vi "GetHight.vi"(8 "error in (no error)":errorcluster, 11 "Triangle in":refnum<class "Triangle.lvclass">) -> (0 "error out":errorcluster, 2 "Hight":i16, 3 "Triangle out":refnum<class "Triangle.lvclass">)   [LabVIEW 2021, in "Picture2D.lvlib" / "Triangle.lvclass"]
uses:
  Triangle.lvclass
  Triangle.lvclass/Triangle.ctl
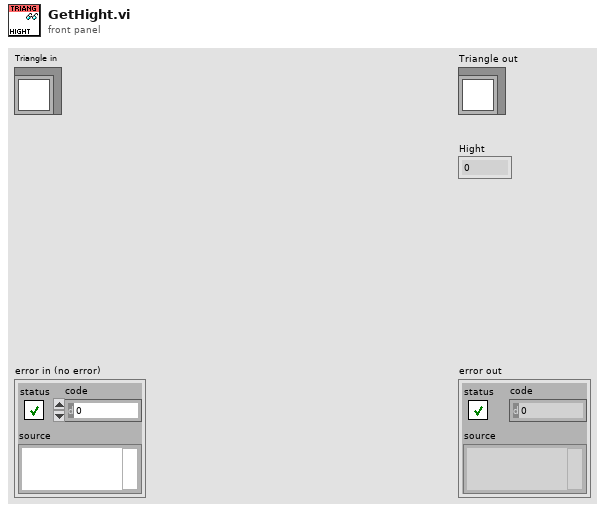
[diagram p1: front panel]
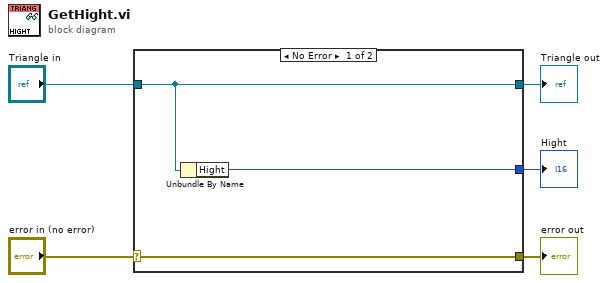
[diagram p0: block diagram]
diagram:
  n1 = case shown="No Error" "error in (no error)" {
    selector: "error in (no error)" -> [w8 w9]
    tunnel: [w8 w9] -> w4
    tunnel: [w7 w10] -> w2
    tunnel: "Triangle in" -> [w7 w10]
    tunnel: [w6 _] -> w1
    frame No Error {
      n2 = Unbundle By Name(w7) -> ("Hight"=w6:i16)
    }
    frame Error {
    }
  }
  "error out" <- w4
  "Triangle out" <- w2
  "Hight" <- w1
